vi "Degrees to Radians.vi"   [LabVIEW 2020, in "NI_AngleConversion.lvlib"]
doc: "Converts data from degrees to radians."
uses:
  <vilib>/Analysis/NI_AngleConversion.lvlib
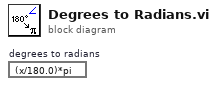
[diagram p0: block diagram]
diagram:
  n1 = expression code="(x/180.0)*pi" "degrees to radians"() -> ()  [unwired: 1 in, 1 out]
